vi "Build State.vi"(8 "error in":errorcluster, 11 "Data in":T2={"Class"={"Ants"=refnum, "Layer"=refnum, "Templates"=refnum, "Icon"=refnum, "Glyph"=refnum, "Settings"=refnum, "Tools"=refnum, "History"=refnum}, "Ref"={"Add Layer"=refnum, "Remove Layer"=refnum, "Line Text"=[], "Body Text Spec"=refnum, "DNL_Font"=refnum, "glyph path str"=refnum, "templates path str"=refnum, "Arrow Up"=refnum, "Arrow Down"=refnum, "IE VI Ref"=refnum, "Glyphs tree"=refnum, "Templates tree"=refnum, "Layer Icon Text"=refnum, "Layer Template"=refnum, "Body Text"=refnum, "Search Templates"=refnum, "TextMarker"=refnum, "Tab Control"=refnum, "Search Glyphs"=refnum, "Line Color"=refnum, "DNL_Glyphs []"=refnum, "Fill Color"=refnum, "Tools"=refnum, "Icon"=refnum, "Preview"=refnum, "Ants"=refnum, "Terminals"=refnum, "menu reference"=refnum, "LayerNames"=[], "GlyphLoadAnimation"=refnum, "TemplateLoadAnimation"=refnum, "refreshGlyphs"=refnum, "refreshTemplates"=refnum}, "Support"={"AntsRect"={"left"=0, "top"=0, "right"=0, "bottom"=0}, "Mouse Move Coords"={"Horizontal"=0, "Vertical"=0}, "Mouse Down Coords"={"Horizontal"=0, "Vertical"=0}, "Temp Coord"={"Horizontal"=0, "Vertical"=0}, "Action"=enum."Default", "Edge Color"=4914962, "Fill Color"=16860, "Mouse Down?"=FALSE, "Draft Mode?"=FALSE, "Temp Icon"=bytes[3102], "CTRL Pressed"=FALSE, "Move Selection?"=FALSE, "AntsRect Orig"={"left"=0, "top"=0, "right"=0, "bottom"=0}, "Text"="", "TM Set?"=FALSE, "Mouse inside icon?"=FALSE, "Tool (old value)"=0, "Pencil Move Color"=0, "Swap Colors?"=FALSE, "Shift pressed?"=FALSE}}) -> (0 "error out":errorcluster, 2 "State":T1)   [LabVIEW 2020, in "lv_icon.lvlib" / "History.lvlib"]
doc: "Builds up the state from specific values and references in the global data."
uses:
  History.lvlib
  State.ctl
  vi.lib/LabVIEW Icon API/lv_icon/Classes/Icon/Icon.lvclass
  Class/FakedArray/FakedArray.lvclass
  <vilib>/Utility/miscctls.llb/LVPoint32TypeDef.ctl
  Controls/SupportClass_Action.ctl
  vi.lib/LabVIEW Icon API/lv_icon/Controls/IEColor.ctl
  Controls/Support Cluster.ctl
  lv_icon.lvlib
  Controls/References Cluster.ctl
  Class/Tools/Tools Paint.lvclass
  Class/Settings/Settings.lvclass
  Class/Icon Library/Glyph.lvclass
  Class/Ants/Ants.lvclass
  History/History.lvclass
  Controls/IE Classes.ctl
  Controls/Global Data.ctl
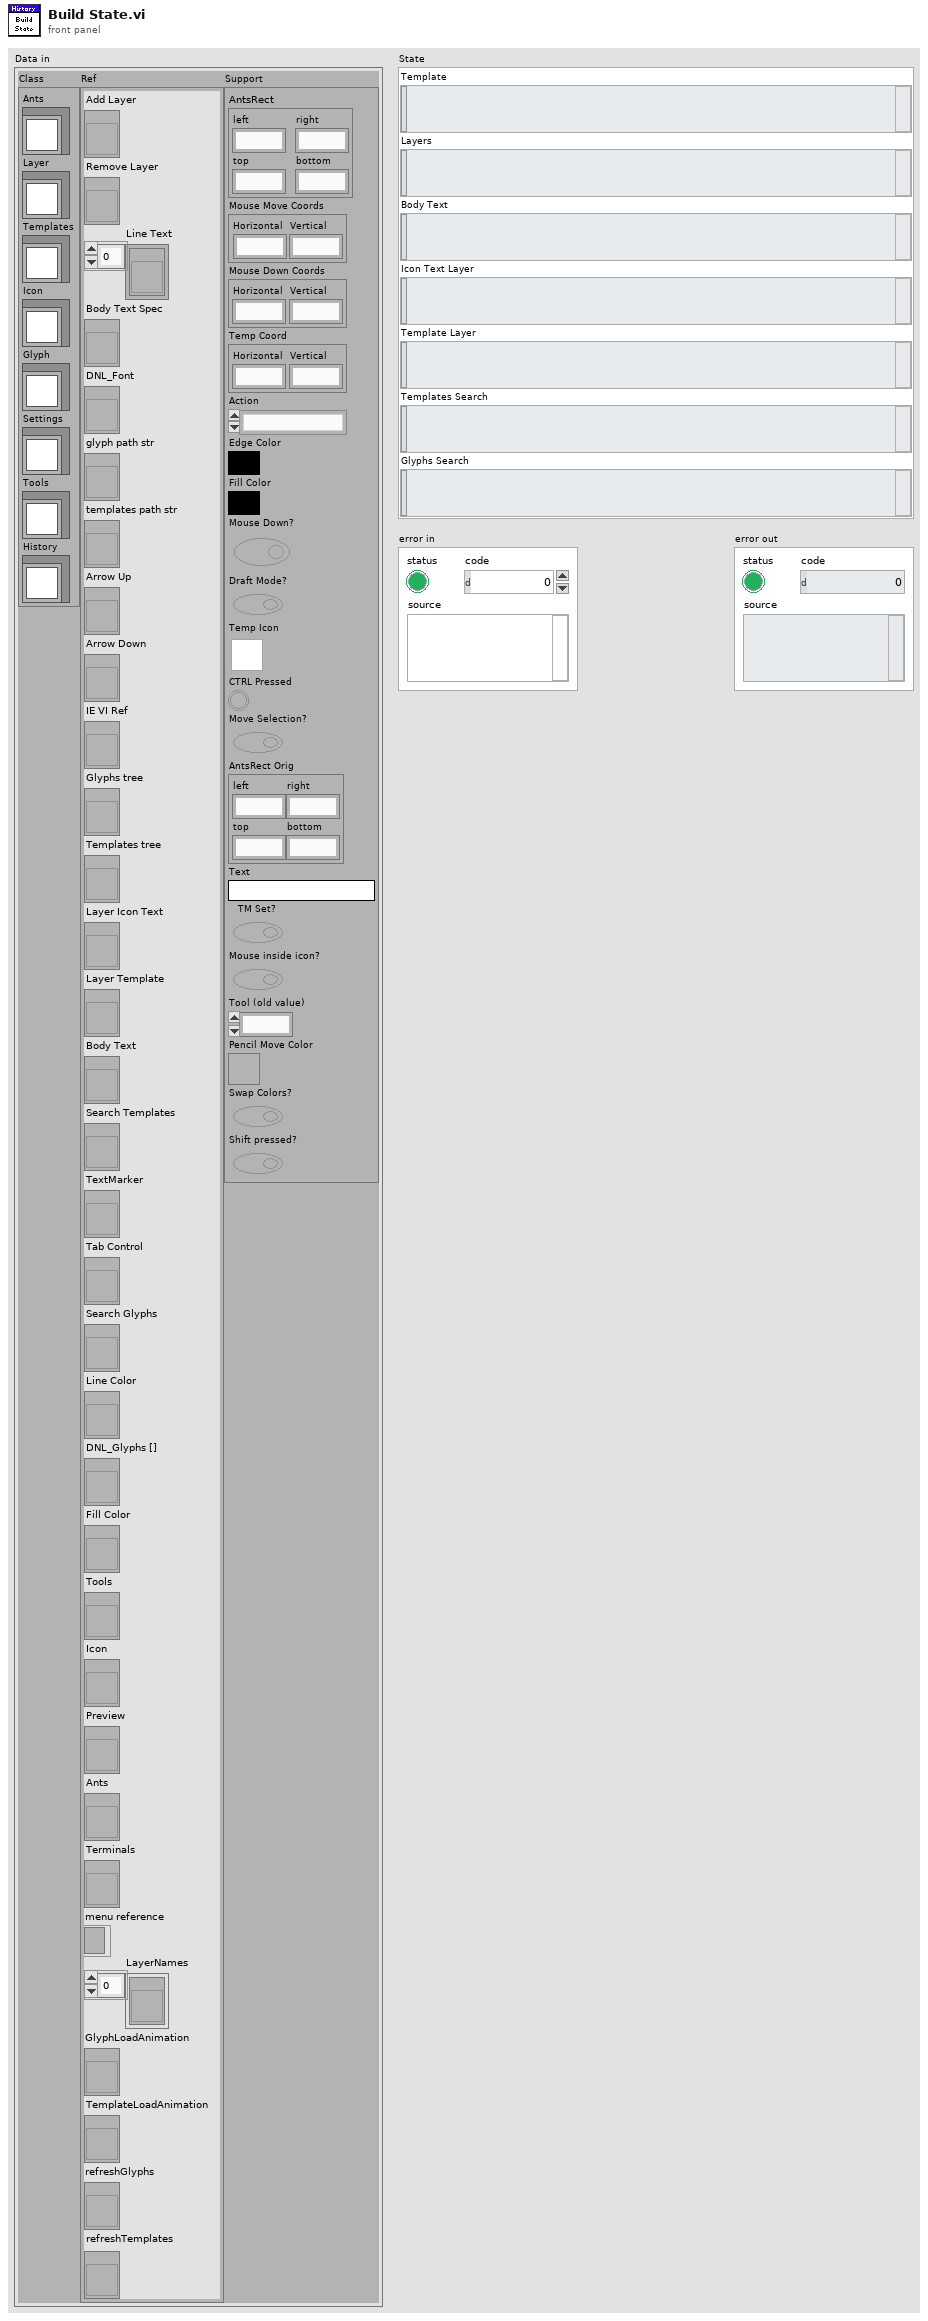
[diagram p1: front panel]
types:
  T1 = typedef "lv_icon.lvlib/History.lvlib/State.ctl" = cluster{"Template":string, "Layers":string, "Body Text":string, "Icon Text Layer":string, "Template Layer":string, "Templates Search":string, "Glyphs Search":string}
  T2 = typedef "lv_icon.lvlib/Global Data.ctl" = cluster{"Class":T3, "Ref":T4, "Support":T5}
  T3 = typedef "lv_icon.lvlib/IE Classes.ctl" = cluster{"Ants":refnum<class "Ants.lvclass">, "Layer":refnum<class "FakedArray.lvclass">, "Templates":refnum<class "FakedArray.lvclass">, "Icon":refnum<class "Icon.lvclass">, "Glyph":refnum<class "Glyph.lvclass">, "Settings":refnum<class "Settings.lvclass">, "Tools":refnum<class "Tools Paint.lvclass">, "History":refnum<class "History.lvclass">}
  T4 = typedef "lv_icon.lvlib/References Cluster.ctl" = cluster{"Add Layer":refnum<vi>, "Remove Layer":refnum<vi>, "Line Text":refnum<vi>[], "Body Text Spec":refnum<vi>, "DNL_Font":refnum<vi>, "glyph path str":refnum<vi>, "templates path str":refnum<vi>, "Arrow Up":refnum<vi>, "Arrow Down":refnum<vi>, "IE VI Ref":refnum<vi>, "Glyphs tree":refnum<vi>, "Templates tree":refnum<vi>, "Layer Icon Text":refnum<vi>, "Layer Template":refnum<vi>, "Body Text":refnum<vi>, "Search Templates":refnum<vi>, "TextMarker":refnum<vi>, "Tab Control":refnum<vi>, "Search Glyphs":refnum<vi>, "Line Color":refnum<vi>, "DNL_Glyphs []":refnum<vi>, "Fill Color":refnum<vi>, "Tools":refnum<vi>, "Icon":refnum<vi>, "Preview":refnum<vi>, "Ants":refnum<vi>, "Terminals":refnum<vi>, "menu reference":refnum<k9>, "LayerNames":refnum<vi>[], "GlyphLoadAnimation":refnum<vi>, "TemplateLoadAnimation":refnum<vi>, "refreshGlyphs":refnum<vi>, "refreshTemplates":refnum<vi>}
  T5 = typedef "lv_icon.lvlib/Support Cluster.ctl" = cluster{"AntsRect":cluster{"left":i16, "top":i16, "right":i16, "bottom":i16}, "Mouse Move Coords":T6, "Mouse Down Coords":T6, "Temp Coord":T6, "Action":T7, "Edge Color":T8, "Fill Color":T8, "Mouse Down?":bool, "Draft Mode?":bool, "Temp Icon":picture, "CTRL Pressed":bool, "Move Selection?":bool, "AntsRect Orig":cluster{"left":i16, "top":i16, "right":i16, "bottom":i16}, "Text":string, "TM Set?":bool, "Mouse inside icon?":bool, "Tool (old value)":u32, "Pencil Move Color":u32, "Swap Colors?":bool, "Shift pressed?":bool}
  T6 = typedef "LVPoint32TypeDef.ctl" = cluster{"Horizontal":i32, "Vertical":i32}
  T7 = typedef "SupportClass_Action.ctl" = enum16{"Default", "Move Selection", "Glyph Library", "Tool"}
  T8 = typedef "IEColor.ctl" = u32
  T9 = cluster{"LayerIcon":picture, "LayerName":string, "Opacity":u8, "Visibility?":bool}
  T10 = typedef "Font.ctl" = string
  T11 = typedef "Alignment.ctl" = u16
  T12 = typedef "Font Size.ctl" = u8
  T13 = cluster{"Line 1 text":string, "Line 2 text":string, "Line 3 text":string, "Line 4 text":string, "Line 1 color":u32, "Line 2 color":u32, "Line 3 color":u32, "Line 4 color":u32, "Body Text Spec":cluster{"DNL_Font":T10, "Alignment":T11, "Size":T12}, "Center text vertically":bool, "Capitalize Text":bool}
  T14 = typedef "Graphic.ctl" = cluster{"Rectangle":cluster{"left":i16, "top":i16, "right":i16, "bottom":i16}, "Path":path, "Image":picture, "Filter":string, "FileName":string}
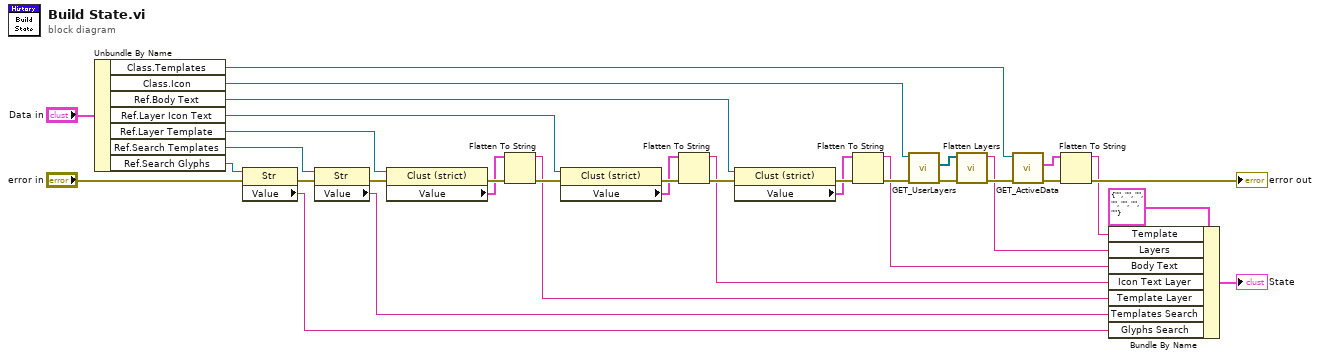
[diagram p0: block diagram]
diagram:
  n1 = Unbundle By Name("Data in") -> ("Class.Templates"=w3:refnum<class "FakedArray.lvclass">, "Class.Icon"=w14:refnum<class "Icon.lvclass">, "Ref.Body Text"=w16:refnum<vi>, "Ref.Layer Icon Text"=w17:refnum<vi>, "Ref.Layer Template"=w18:refnum<vi>, "Ref.Search Templates"=w19:refnum<vi>, "Ref.Search Glyphs"=w20:refnum<vi>)
  n2 = property class="Str"(reference=w20, error in="error in") -> (error out=w34:errorcluster, "Value"=w10:string)  [unwired: 1 out]
  n3 = property class="Str"(reference=w19, error in=w34) -> (error out=w35:errorcluster, "Value"=w9:string)  [unwired: 1 out]
  n4 = property class="Clust (strict)"(reference=w18, error in=w35) -> (error out=w31:errorcluster, "Value"=w13:T9)  [unwired: 1 out]
  n5 = Flatten To String(anything=w13, error in (no error)=w31) -> (data string=w8:string, error out=w30:errorcluster)  [unwired: 3 out]
  n6 = property class="Clust (strict)"(reference=w17, error in=w30) -> (error out=w29:errorcluster, "Value"=w12:T9)  [unwired: 1 out]
  n7 = Flatten To String(anything=w12, error in (no error)=w29) -> (data string=w7:string, error out=w28:errorcluster)  [unwired: 3 out]
  n8 = property class="Clust (strict)"(reference=w16, error in=w28) -> (error out=w27:errorcluster, "Value"=w11:T13)  [unwired: 1 out]
  n9 = Flatten To String(anything=w11, error in (no error)=w27) -> (data string=w6:string, error out=w26:errorcluster)  [unwired: 3 out]
  n10 = call-dynamic "GET_UserLayers.vi"("error in (no error)"=w26, "Icon.lvclass in"=w14) -> ("error out"=w32:errorcluster, "All Layers"=w15:refnum<class "Layer.lvclass">[])  [unwired: 8 out]
  n11 = call "Flatten Layers.vi"("Error In"=w32, "Layers"=w15) -> ("Error Out"=w25:errorcluster, "String"=w5:string)  [unwired: 8 in]
  n12 = call-dynamic "GET_ActiveData.vi"("error in (no error)"=w25, "FakedArray in"=w3) -> ("error out"=w24:errorcluster, "Path & Icon"=w4:T14)  [unwired: 8 out]
  n13 = Flatten To String(anything=w4, error in (no error)=w24) -> (data string=w2:string, error out=→"error out":errorcluster)  [unwired: 3 out]
  n14 = Bundle By Name(cluster=T1 {"Template"="", "Layers"="", "Body Text"="", "Icon Text Layer"="", "Template Layer"="", "Templates Search"="", "Glyphs Search"=""} ("State"), "Template"=w2, "Layers"=w5, "Body Text"=w6, "Icon Text Layer"=w7, "Template Layer"=w8, "Templates Search"=w9, "Glyphs Search"=w10) -> (→"State":T1)
